vi "LogRelayError.vi"(0 "Path":path, 7 "GuiderRA Error":errorcluster, 11 "GuiderDEC Error":errorcluster) -> ()   [LabVIEW 2019]
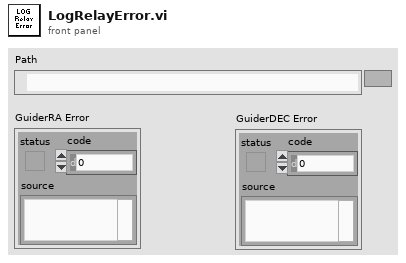
[diagram p1: front panel]
types:
  T1 = enum16{"open", "replace", "create", "open or create", "replace or create", "replace or create with confirmation"}
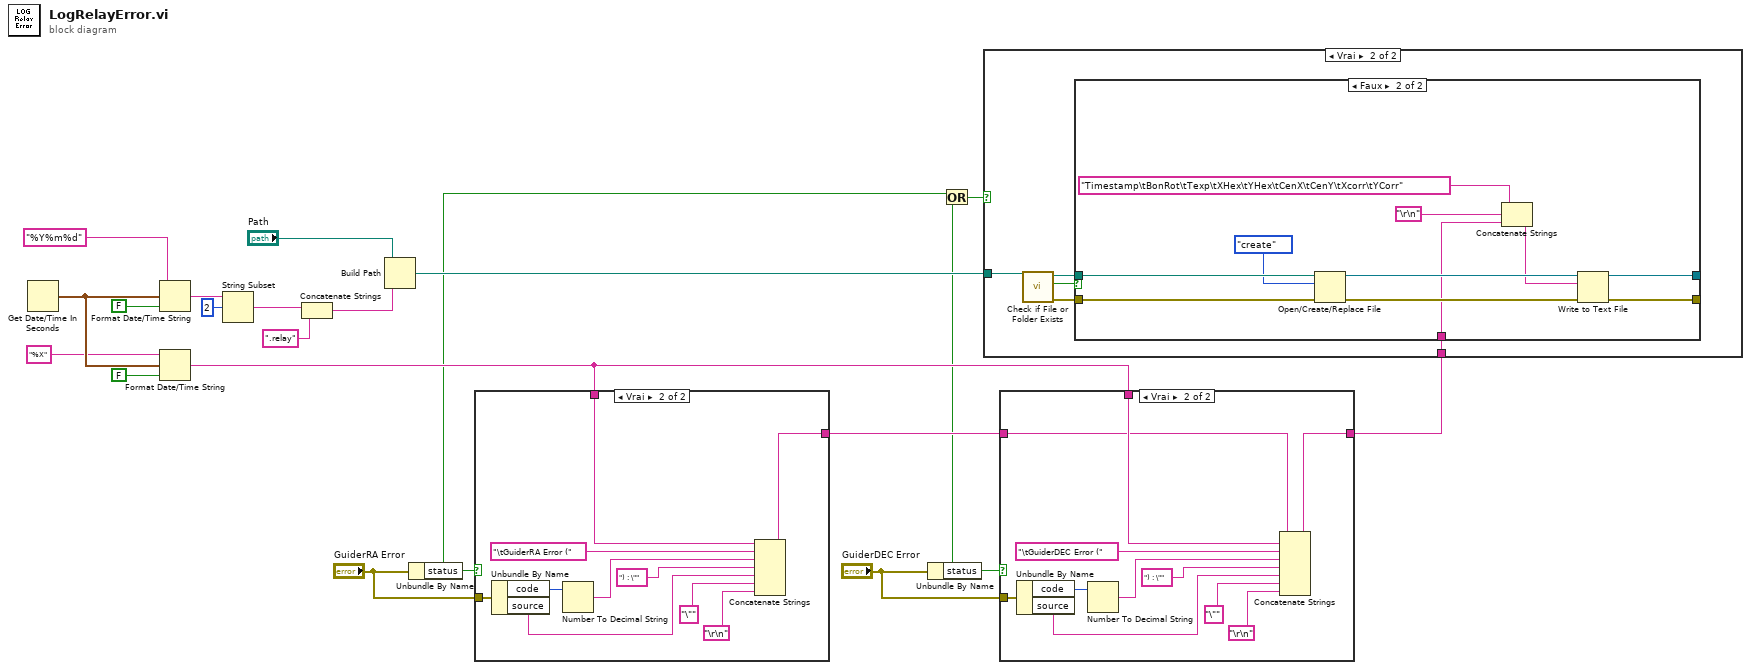
[diagram p0: block diagram]
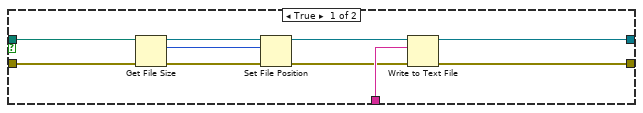
[diagram p3: hidden frame]
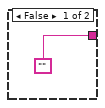
[diagram p5: hidden frame]
diagram:
  n1 = Get Date/Time In Seconds() -> (seconds since 1Jan1904=w19:timestamp)
  n2 = Format Date/Time String(time format string (%c)="%Y%m%d", seconds (now)=w19, UTC format=FALSE) -> (date/time string=w15:string)
  n3 = Format Date/Time String(time format string (%c)="%X", seconds (now)=w19, UTC format=FALSE) -> (date/time string=w4:string)
  n4 = String Subset(string=w15, offset (0)=2) -> (substring=w12:string)  [unwired: 1 in]
  n5 = Concatenate Strings(w12, ".relay" ("string")) -> (w10:string)
  n6 = Build Path(base path="Path", name or relative path=w10) -> (appended path=w5:path)
  n7 = Unbundle By Name("GuiderRA Error") -> ("status"=w1:bool)
  n8 = case shown="Vrai" w1 {
    tunnel: "GuiderRA Error" -> [_ w31]
    tunnel: ["" w23] -> w7
    tunnel: w4 -> [_ w22]
    frame False {
    }
    frame True {
      n9 = Unbundle By Name(w31) -> ("code"=w30:i32, "source"=w26:string)
      n10 = Number To Decimal String(number=w30) -> (decimal integer string=w29:string)  [unwired: 1 in]
      n11 = Concatenate Strings(w22, "\tGuiderRA Error (", w29, ") : \"", w26, "\"", "\r\n") -> (w23:string)
    }
  }
  n12 = Unbundle By Name("GuiderDEC Error") -> ("status"=w2:bool)
  n13 = Or(x=w1, y=w2) -> (x .or. y?=w3:bool)
  n14 = case shown="Vrai" w2 {
    tunnel: w7 -> [w32 w33]
    tunnel: "GuiderDEC Error" -> [_ w43]
    tunnel: [w32 w35] -> w6
    tunnel: w4 -> [_ w34]
    frame False {
    }
    frame True {
      n15 = Unbundle By Name(w43) -> ("code"=w42:i32, "source"=w38:string)
      n16 = Number To Decimal String(number=w42) -> (decimal integer string=w41:string)  [unwired: 1 in]
      n17 = Concatenate Strings(w33, w34, "\tGuiderDEC Error (", w41, ") : \"", w38, "\"", "\r\n") -> (w35:string)
    }
  }
  n18 = case shown="Vrai" w3 {
    tunnel: w6 -> [_ w45]
    tunnel: w5 -> [_ w44]
    frame False {
    }
    frame True {
      n19 = call <vilib>:"Check if File or Folder Exists.vi"("path"=w44) -> ("error out"=w48:errorcluster, "file or folder exists?"=w46:bool, "dup path"=w47:path)  [unwired: 8 in]
      n20 = case shown="Faux" w46 {
        tunnel: w47 -> [w52 w69]
        tunnel: w48 -> [w51 w68]
        tunnel: [w58 w67] -> _
        tunnel: [w57 w66] -> _
        tunnel: w45 -> [w56 w60]
        frame True {
          n21 = Get File Size(file=w52, error in=w51) -> (refnum out=w55:refnum<file>, size (in bytes)=w54:i64, 0:w53:errorcluster)
          n22 = Set File Position(offset (in bytes) (0)=w54, refnum=w55, error in=w53) -> (refnum out=w50:refnum<file>, error out=w49:errorcluster)  [unwired: 1 in]
          n23 = Write to Text File(file (use dialog)=w50, text=w56, error in=w49) -> (refnum out=w58:refnum<file>, error out=w57:errorcluster)  [unwired: 1 in, 1 out]
        }
        frame False {
          n24 = Open/Create/Replace File(file path (use dialog)=w69, error in=w68, operation (0:open)=T1."create") -> (refnum out=w64:refnum<file>, error out=w63:errorcluster)  [unwired: 3 in, 1 out]
          n25 = Concatenate Strings("Timestamp\tBonRot\tTexp\tXHex\tYHex\tCenX\tCenY\tXcorr\tYCorr", "\r\n", w60) -> (w59:string)
          n26 = Write to Text File(file (use dialog)=w64, text=w59, error in=w63) -> (refnum out=w67:refnum<file>, error out=w66:errorcluster)  [unwired: 1 in, 1 out]
        }
      }
    }
  }
